vi "ThrustTest.vi"() -> ()   [LabVIEW 2015]
uses:
  VI Files/StateMachineControl.ctl
  Classes/Scale/OHAUS AV8101/OHAUS AV8101.lvclass
  Classes/Scale/Scale Emulator/Scale Emulator.lvclass
  Classes/Ammeter/ACS759/ACS759.lvclass
  Classes/Ammeter/Ammeter Emulator/Ammeter Emulator.lvclass
  Classes/ESC/Detrum12A/Dectrum12A.lvclass
  Classes/ESC/ESC Emulator/ESC Emulator.lvclass
  Classes/ESC/Exceed RC Volcano Series/Exceed RC Volcano Series.lvclass
  <vilib>/express/express shared/transition.llb/Dynamic To Waveform Array.vi
  <vilib>/express/express signal manip/GetorSetDDTAttributes/Set DDT Attributes/SetT0.vi
  <vilib>/express/express shared/transition.llb/Waveform Array To Dynamic.vi
  <vilib>/express/express signal manip/GetorSetDDTAttributes/Set DDT Attributes/Set DDT Properties.xnode
  Classes/Scale/Scale.lvclass
  Classes/ESC/ESC.lvclass
  Classes/Ammeter/Ammeter.lvclass
panel:
  out "Save Location":path caption="selected path"
  in  "Scale Model":enum16{"OHAUS AV8101", "Emulator"}(ring)=enum."Emulator"
  in  "Ammeter Model":enum16{"ACS759", "Emulator"}(ring)=enum."Emulator"
  in  "ESC Model":T1(ring)=enum."Emulator"
  in  "Stabilize Time [ms]":u32=5000
  in  "Throttle % Increment":dbl=10.0
  in  "State":T2
  out "Thrust vs. Amp Draw Curve":cluster{dbl[], dbl[]}(graph)
  in  "Exit":bool
  in  "Run Test":bool
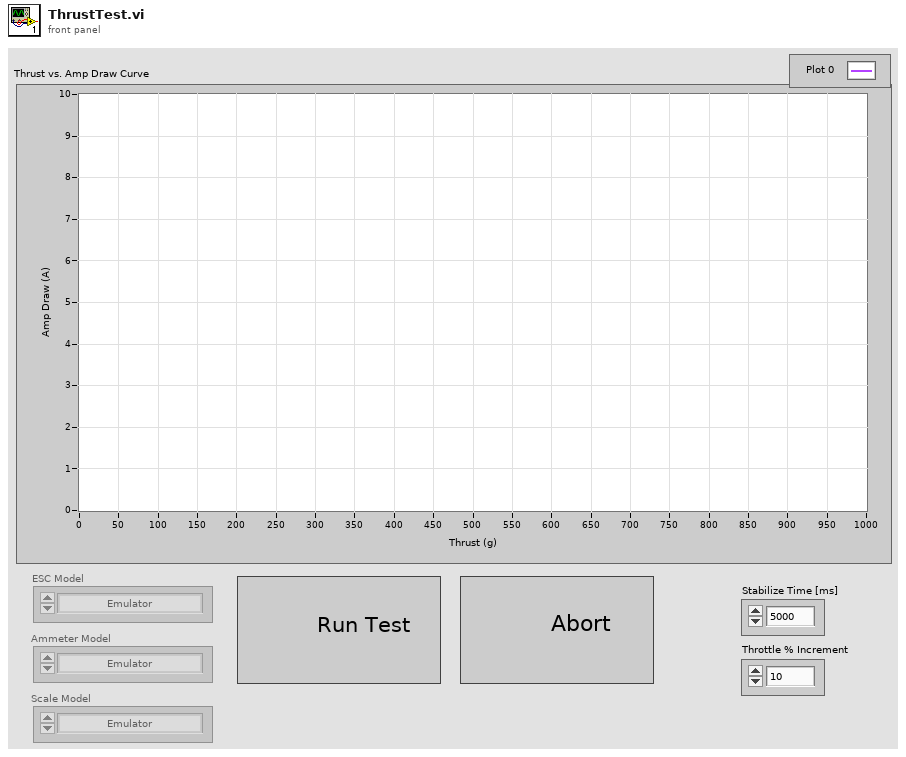
[diagram p1: front panel]
types:
  T1 = enum16{"Detrum 12A", "Emulator", "ExceedRC Volcano Series"}
  T2 = typedef "StateMachineControl.ctl" = enum16{"Wait for Go", "First Signal", "Wait to Stabilize ", "Record XY", "Increment Signal", "Wait for Save", "Save"}
  T3 = enum8{"Enabled", "Disabled", "Disabled and Grayed Out"}
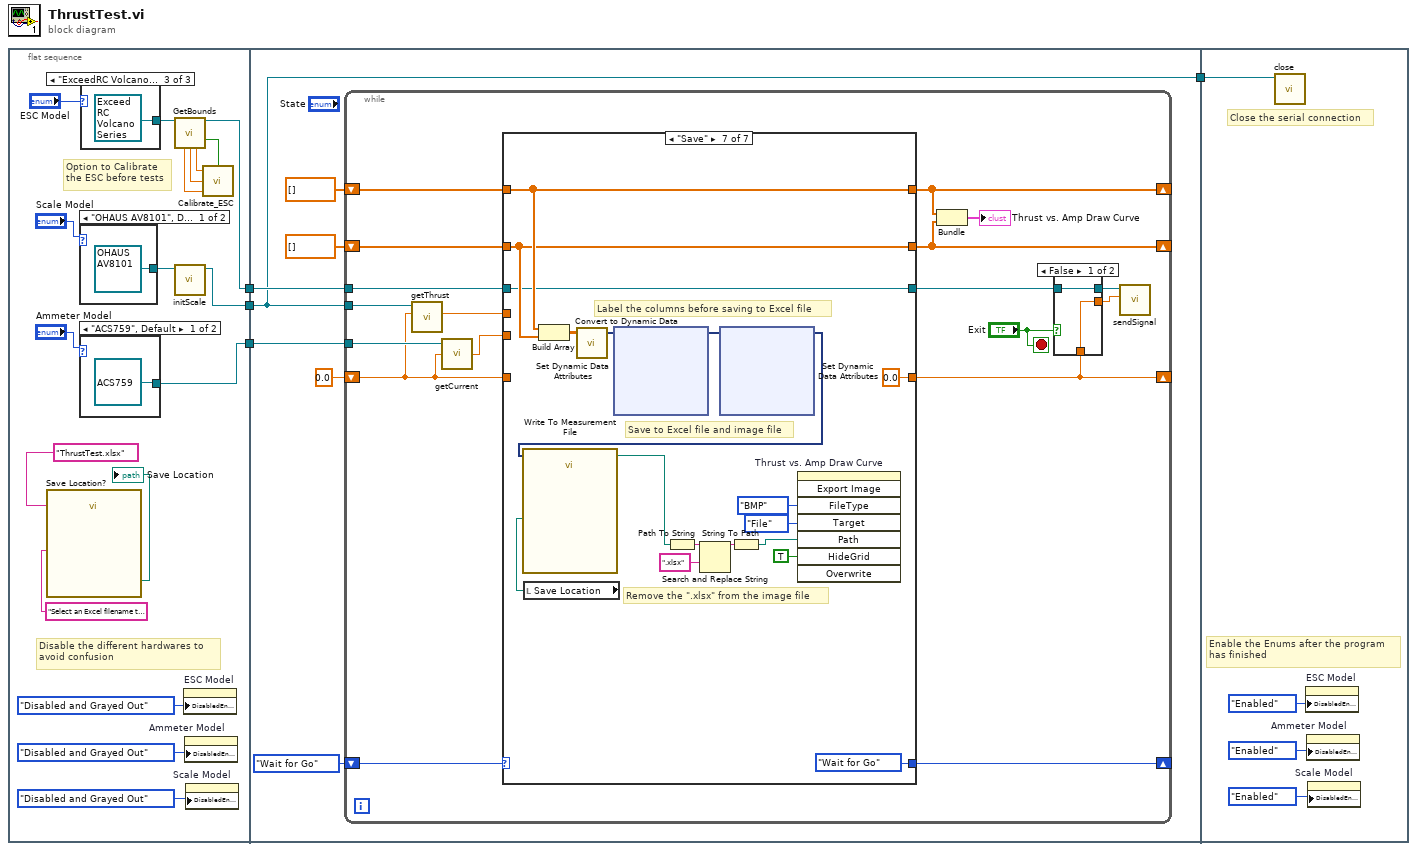
[diagram p0: block diagram]
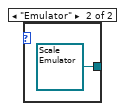
[diagram p2: hidden frame]
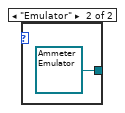
[diagram p3: hidden frame]
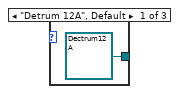
[diagram p4: hidden frame]
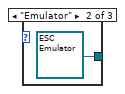
[diagram p5: hidden frame]
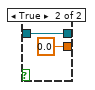
[diagram p6: hidden frame]
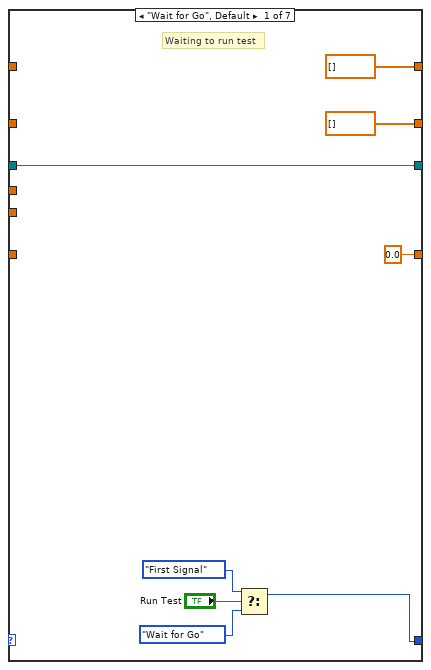
[diagram p7: hidden frame]
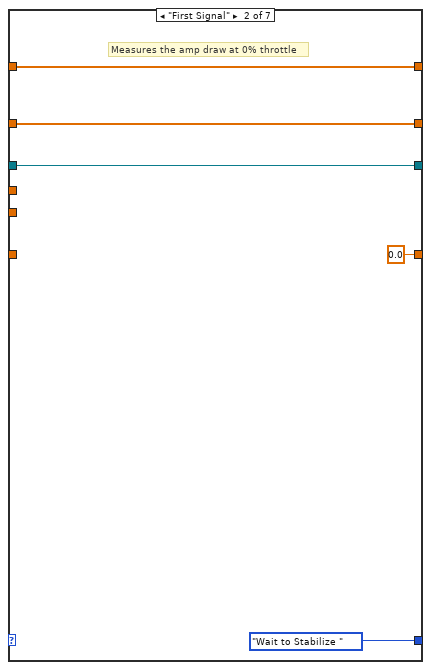
[diagram p8: hidden frame]
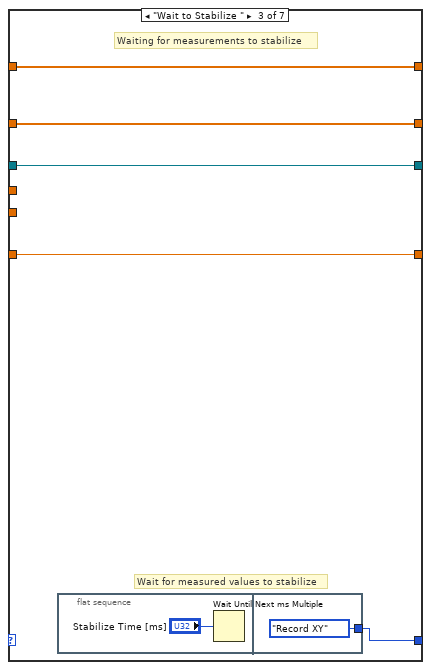
[diagram p9: hidden frame]
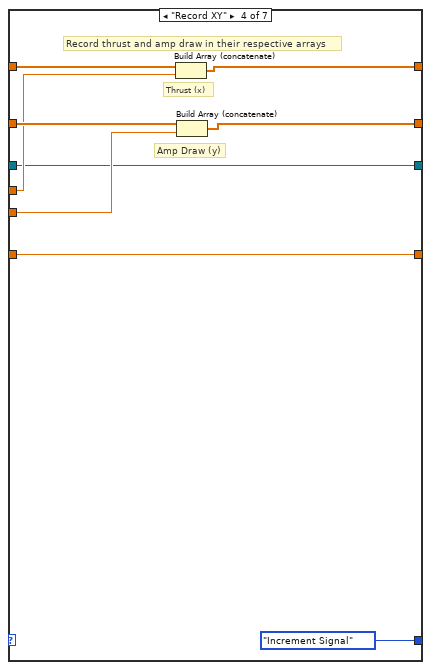
[diagram p10: hidden frame]
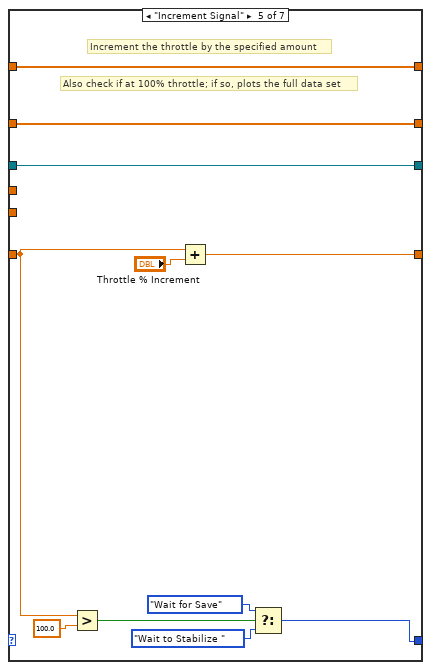
[diagram p11: hidden frame]
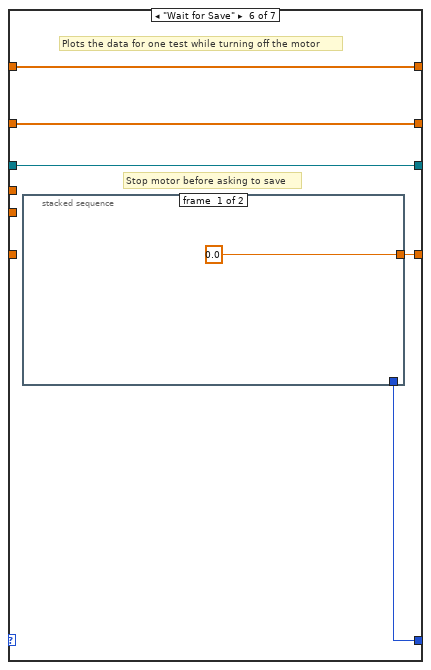
[diagram p12: hidden frame]
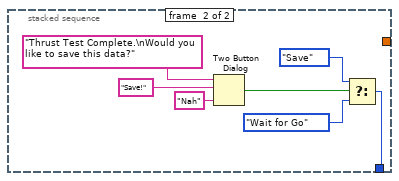
[diagram p13: hidden frame]
diagram:
  n1 = flat-sequence {
    tunnel: [w16] -> w4
    tunnel: [w14] -> w3
    tunnel: [w8] -> w2
    tunnel: w4 -> [w32]
    tunnel: w3 -> [w31]
    tunnel: w2 -> [w30]
    tunnel: [w30] -> w1
    tunnel: w1 -> [w166]
    frame #0 {
      # "Disable the different hardwares to \navoid confusion"
      # "Option to Calibrate\nthe ESC before tests"
      n2 = call "Save Location?"("prompt"="Select an Excel filename to save data in (Convention \"Filename.xlsx\") **INCLUDING THE .xlsx IS REQUIRED**", "default name"="ThrustTest.xlsx") -> ("selected path"=→"Save Location":path)  [unwired: 10 in, 3 out]
      n3 = case shown="\"OHAUS AV8101\", Default" "Scale Model" {
        tunnel: [refnum<class "OHAUS AV8101.lvclass"> refnum ("OHAUS AV8101.lvclass") refnum<class "Scale Emulator.lvclass"> refnum ("Scale Emulator.lvclass")] -> w9
        frame "OHAUS AV8101", Default {
        }
        frame "Emulator" {
        }
      }
      n4 = case shown="\"ACS759\", Default" "Ammeter Model" {
        tunnel: [refnum<class "ACS759.lvclass"> refnum ("ACS759.lvclass") refnum<class "Ammeter Emulator.lvclass"> refnum ("Ammeter Emulator.lvclass")] -> w14
        frame "ACS759", Default {
        }
        frame "Emulator" {
        }
      }
      n5 = case shown="\"ExceedRC Volcano Series\"" "ESC Model" {
        tunnel: [refnum<class "Dectrum12A.lvclass"> refnum ("Dectrum12A.lvclass") refnum<class "ESC Emulator.lvclass"> refnum ("ESC Emulator.lvclass") refnum<class "Exceed RC Volcano Series.lvclass"> refnum ("Exceed RC Volcano Series.lvclass")] -> w20
        frame "Detrum 12A", Default {
        }
        frame "Emulator" {
        }
        frame "ExceedRC Volcano Series" {
        }
      }
      n6 = call-dynamic "GetBounds.vi"("ESC in"=w20) -> ("ESC out"=w16:refnum<class "ESC.lvclass">, "Calibrate?"=w10:bool, "PWM Frequency"=w19:dbl, "Duty Cycle Min"=w18:dbl, "Duty Cycle Max"=w17:dbl)  [unwired: 9 in, 1 out]
      n7 = call-dynamic "initScale.vi"("Scale in"=w9) -> ("Scale out"=w8:refnum<class "Scale.lvclass">)  [unwired: 9 in, 1 out]
      n8 = property on="ESC Model" class="Enum (strict)"("DisabledEnum"=T3."Disabled and Grayed Out" ("Disabled")) -> ()  [unwired: 2 in, 2 out]
      n9 = property on="Ammeter Model" class="Enum (strict)"("DisabledEnum"=T3."Disabled and Grayed Out" ("Disabled")) -> ()  [unwired: 2 in, 2 out]
      n10 = property on="Scale Model" class="Enum (strict)"("DisabledEnum"=T3."Disabled and Grayed Out" ("Disabled")) -> ()  [unwired: 2 in, 2 out]
      n11 = call "Calibrate_ESC.vi"("Calibrate?"=w10, "PWM Frequency"=w19, "Min Duty Cycle (%)"=w18, "Max Duty Cycle (%)"=w17) -> ()  [unwired: 1 in]
    }
    frame #1 {
      n12 = while {
        shift-right: [w53] -> _
        shift-left: StateMachineControl."Wait for Go" ("State") -> [w54]
        shift-right: [w40] -> _
        shift-left: 0.0 ("PWM Increment") -> [w43]
        shift-right: [w50] -> _
        shift-left: dbl[] [] -> [w52]
        shift-right: [w49] -> _
        shift-left: dbl[] [] -> [w51]
        tunnel: w32 -> [w48]
        tunnel: w31 -> [w47]
        tunnel: w30 -> [w45]
        stop <- "Exit" stop-if-true
        n13 = call-dynamic "getThrust.vi"("Throttle % [0-100]"=w43, "Scale in"=w45) -> ("Thrust [g]"=w44:dbl)  [unwired: 7 in, 2 out]
        n14 = call-dynamic "getCurrent.vi"("Throttle % [0-100]"=w43, "Ammeter in"=w47) -> ("Current [Amps]"=w46:dbl)  [unwired: 1 in, 2 out]
        n15 = case shown="\"Save\"" w54 {
          tunnel: [w63 StateMachineControl."Wait to Stabilize " ("State") w76 StateMachineControl."Increment Signal" ("State") w91 w99 StateMachineControl."Wait for Go" ("State")] -> w53
          tunnel: w52 -> [_ w69 w74 w87 w96 w102 w129]
          tunnel: w51 -> [_ w70 w75 w86 w97 w103 w128]
          tunnel: [dbl[] [] w70 w75 w85 w97 w103 w128] -> w49
          tunnel: [dbl[] [] w69 w74 w84 w96 w102 w129] -> w50
          tunnel: [0.0 ("PWM Increment") 0.0 ("PWM Increment") w73 w80 w98 w100 0.0 ("PWM Increment")] -> w40
          tunnel: w43 -> [_ _ w73 w80 w90 _ _]
          tunnel: w44 -> [_ _ _ w82 _ _ _]
          tunnel: w46 -> [_ _ _ w81 _ _ _]
          tunnel: [w59 w67 w72 w79 w88 w101 w125] -> w42
          tunnel: w48 -> [w59 w67 w72 w79 w88 w101 w125]
          frame "Wait for Go", Default {
            # "Waiting to run test"
            n16 = Select(t=StateMachineControl."First Signal" ("State"), s="Run Test", f=StateMachineControl."Wait for Go" ("State")) -> (s? t:f=w63:T2)
          }
          frame "First Signal" {
            # "Measures the amp draw at 0% throttle"
          }
          frame "Wait to Stabilize " {
            # "Waiting for measurements to stabilize"
            # "Wait for measured values to stabilize"
            n17 = flat-sequence {
              tunnel: [StateMachineControl."Record XY" ("State")] -> w76
              frame #0 {
                n18 = Wait Until Next ms Multiple(millisecond multiple="Stabilize Time [ms]") -> ()  [unwired: 1 out]
              }
              frame #1 {
              }
            }
          }
          frame "Record XY" {
            # "Record thrust and amp draw in their respective arrays"
            # "Amp Draw (y)"
            # "Thrust (x)"
            n19 = Build Array (concatenate)(w87, w82) -> (w84:dbl[])
            n20 = Build Array (concatenate)(w86, w81) -> (w85:dbl[])
          }
          frame "Increment Signal" {
            # "Also check if at 100% throttle; if so, plots the full data set"
            # "Increment the throttle by the specified amount"
            n21 = Greater?(x=w90, y=100.0) -> (0:w94:bool)
            n22 = Add(x=w90, y="Throttle % Increment") -> (x+y=w98:dbl)
            n23 = Select(t=StateMachineControl."Wait for Save" ("State"), s=w94, f=StateMachineControl."Wait to Stabilize " ("State")) -> (s? t:f=w91:T2)
          }
          frame "Wait for Save" {
            # "Stop motor before asking to save"
            # "Plots the data for one test while turning off the motor"
            n24 = stacked-sequence {
              tunnel: [0.0 ("PWM Increment") _] -> w100
              tunnel: [_ w105] -> w99
              frame #0 {
              }
              frame #1 {
                n25 = Two Button Dialog(message="Thrust Test Complete.\nWould you like to save this data?", 1:"Nah" ("F button name (\"Cancel\")"), 2:"Save!" ("T button name (\"OK\")")) -> (T button?=w111:bool)
                n26 = Select(t=StateMachineControl."Save" ("State"), s=w111, f=StateMachineControl."Wait for Go" ("State")) -> (s? t:f=w105:T2)
              }
            }
          }
          frame "Save" {
            # "Remove the \".xlsx\" from the image file"
            # "Save to Excel file and image file"
            # "Label the columns before saving to Excel file"
            n27 = local read "Save Location"() -> (w120:path)
            n28 = Build Array(w129, w128) -> (w124:dbl[][])
            n29 = call "Convert to Dynamic Data"("2D Array"=w124) -> ("Dynamic Data Type"=w123:dynamicdata)  [unwired: 3 in]
            n30 = xnode "Set Dynamic Data Attributes"("Signals In"=w123) -> ("Signals Out"=w122:dynamicdata)  [unwired: 4 in, 1 out]
            n31 = xnode "Set Dynamic Data Attributes"("Signals In"=w122) -> ("Signals Out"=w121:dynamicdata)  [unwired: 4 in, 1 out]
            n32 = call "Write To Measurement File"("Signals"=w121, "Filename"=w120) -> ("Filename Out"=w112:path)  [unwired: 15 in, 2 out]
            n33 = Path To String(path=w112) -> (string=w116:string)
            n34 = Search and Replace String(input string=w116, search string=".xlsx") -> (result string=w114:string)  [unwired: 6 in, 3 out]
            n35 = String To Path(string=w114) -> (path=w113:path)
            n36 = invoke on="Thrust vs. Amp Draw Curve" class="XYGraph (strict)" method="Export Image"("FileType"=enum32{"BMP", "EPS", "EMF", "PICT"}."BMP" ("File Type"), "Target"=enum32{"File", "Clipboard"}."File", "Path"=w113, "HideGrid"=TRUE ("Hide Grid")) -> ()  [unwired: 4 in, 8 out]
          }
        }
        n37 = Bundle(w50, w49) -> (→"Thrust vs. Amp Draw Curve":cluster{dbl[], dbl[]})  [unwired: 1 in]
        n38 = case shown="False" "Exit" {
          tunnel: [w56 w58] -> w41
          tunnel: w42 -> [w56 w58]
          tunnel: [w55 0.0 ("PWM Increment")] -> w39
          tunnel: w40 -> [w55 _]
          frame False {
          }
          frame True {
          }
        }
        n39 = call-dynamic "sendSignal.vi"("Throttle [%]"=w39, "ESC in"=w41) -> ()  [unwired: 8 in, 2 out]
      }
    }
    frame #2 {
      # "Close the serial connection"
      # "Enable the Enums after the program\nhas finished"
      n40 = call-dynamic "close.vi"("Scale in"=w166) -> ()  [unwired: 9 in, 2 out]
      n41 = property on="ESC Model" class="Enum (strict)"("DisabledEnum"=T3."Enabled" ("Disabled")) -> ()  [unwired: 2 in, 2 out]
      n42 = property on="Ammeter Model" class="Enum (strict)"("DisabledEnum"=T3."Enabled" ("Disabled")) -> ()  [unwired: 2 in, 2 out]
      n43 = property on="Scale Model" class="Enum (strict)"("DisabledEnum"=T3."Enabled" ("Disabled")) -> ()  [unwired: 2 in, 2 out]
    }
  }
